vi "Test Square.vi"() -> ()   [LabVIEW 2015, in "SB SubVIs.lvlib"]
uses:
  SB SubVIs.lvlib
  Type Defs/Action Enum.ctl
  Type Defs/Direction Enum.ctl
  Squares/Shawn/Hail/Hail.lvclass
  Read-Only Globals.vi
  Globals (private).vi
  Square/Square.lvclass
  Type Defs/SB Type Defs.lvlib
panel:
  out "Array 2":T1[](array[typedef])
  out "Array":T2[](array[typedef])
  out "Intensity Graph":i32[][](graph)
  in  "stop":bool
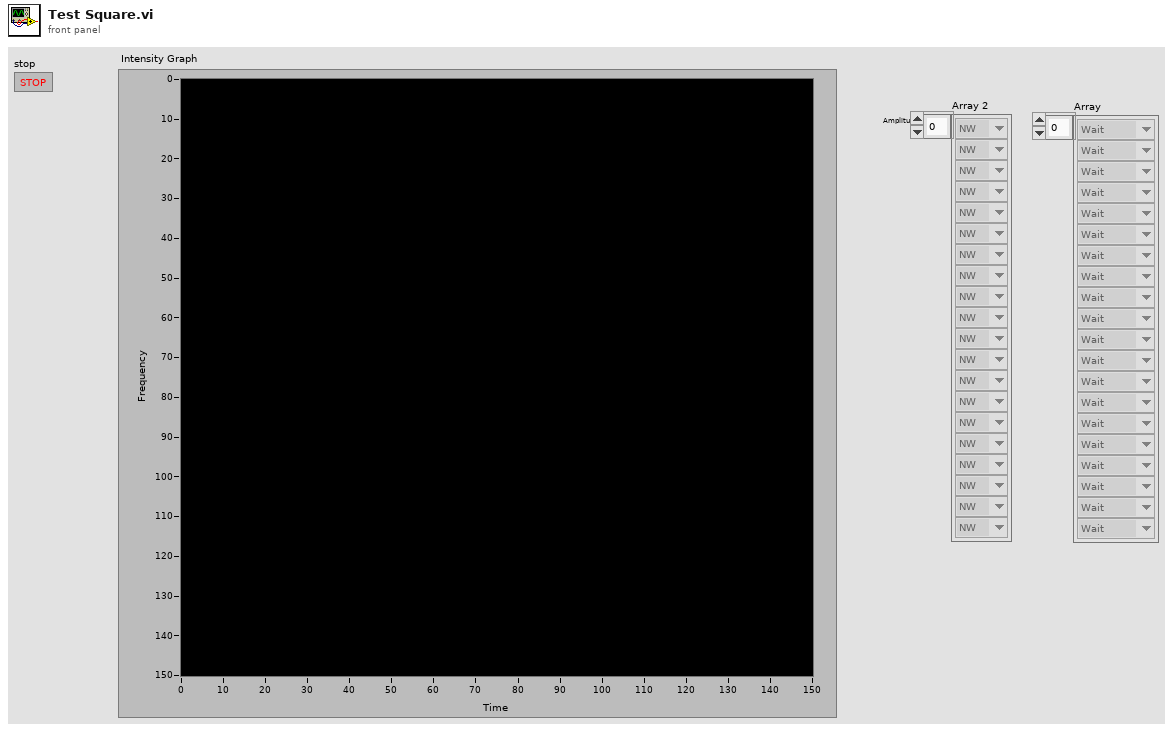
[diagram p1: front panel]
types:
  T1 = typedef "SB Type Defs.lvlib/Direction Enum.ctl" = enum16{"NW", "N", "NE", "E", "SE", "S", "SW", "W"}
  T2 = typedef "SB Type Defs.lvlib/Action Enum.ctl" = enum16{"Wait", "Move", "Attack", "Replicate"}
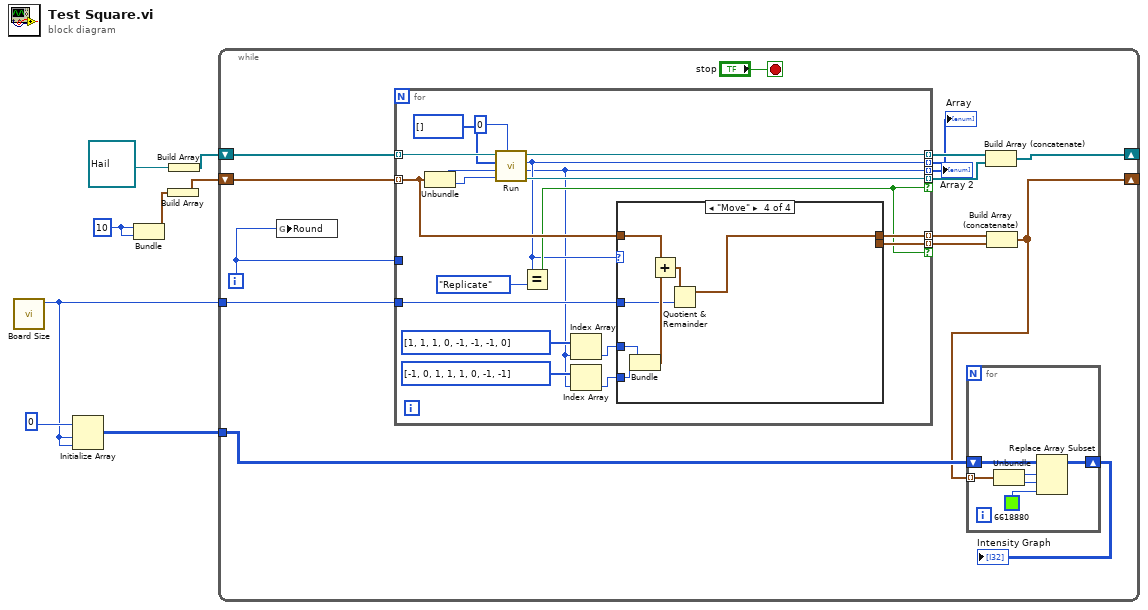
[diagram p0: block diagram]
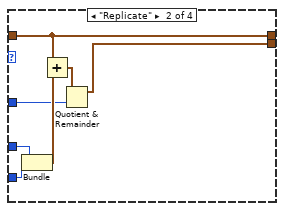
[diagram p3: hidden frame]
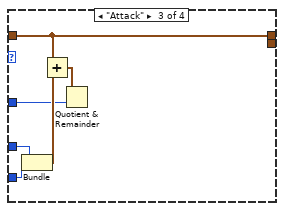
[diagram p4: hidden frame]
diagram:
  w2 = 10
  n1 = call "Board Size.vi"() -> ("Board Size"=w3:i32)  [unwired: 11 in]
  n2 = Initialize Array(0, w3, w3) -> (w1:i32[][])
  n3 = Bundle(w2, w2) -> (w5:cluster{i32, i32})  [unwired: 1 in]
  n4 = Build Array(w5) -> (w6:cluster{i32, i32}[])
  n5 = Build Array(refnum<class "Hail.lvclass"> refnum ("Hail.lvclass")) -> (w8:refnum<class "Hail.lvclass">[])
  n6 = while {
    shift-right: [w20] -> _
    shift-left: w8 -> [w22]
    shift-right: [w11] -> _
    shift-left: w6 -> [w17]
    tunnel: w3 -> [w16]
    tunnel: w1 -> [w13]
    i -> [w23]
    stop <- "stop" stop-if-true
    n7 = global write "Globals (private).vi" "Round"(w23) -> ()
    n8 = for {
      tunnel: w23 -> [_]
      tunnel: w22 -> [w48] mode=indexing
      tunnel: [w47] -> w21 mode=indexing
      tunnel: [w45] -> w19 mode=indexing if=w32
      tunnel: w17 -> [w36] mode=indexing
      tunnel: w16 -> [w34]
      tunnel: [w35] -> w15 mode=indexing
      tunnel: [w33] -> w14 mode=indexing if=w32
      tunnel: [w31] -> w10 mode=indexing
      tunnel: [w30] -> w9 mode=indexing
      n9 = Unbundle(w36) -> (w42:i32, w41:i32)
      n10 = call-dynamic "Run.vi"("Team Index"=0, "Column"=w41, "Row"=w42, "View"=i32[] [], "Square In"=w48) -> ("Replicated"=w45:refnum<class "Square.lvclass">, "Direction"=w30:T1, "Action"=w31:T2, "Square Out"=w47:refnum<class "Square.lvclass">)  [unwired: 3 in]
      n11 = Equal?(x=w31, y=Action_Enum."Replicate") -> (x = y?=w32:bool)
      n12 = Index Array(array=i32[] [1, 1, 1, 0, -1, -1, -1, 0], index=w30) -> (element=w38:i32)
      n13 = Index Array(array=i32[] [-1, 0, 1, 1, 1, 0, -1, -1], index=w30) -> (element=w37:i32)
      n14 = case shown="\"Move\"" w31 {
        tunnel: w38 -> [_ w55 w61 w68]
        tunnel: w37 -> [_ w56 w62 w69]
        tunnel: w36 -> [w49 w51 w57 w63]
        tunnel: [w49 w51 w57 w64] -> w35
        tunnel: w34 -> [_ w52 w58 w65]
        tunnel: [_ w50 _ _] -> w33
        frame "Wait" {
        }
        frame "Replicate" {
          n15 = Bundle("X Loc"=w55, "X Loc"=w56) -> (w54:cluster{"X Loc":i32, "X Loc":i32})  [unwired: 1 in]
          n16 = Add(x=w51, y=w54) -> (x+y=w53:cluster{i32, i32})
          n17 = Quotient & Remainder(x=w53, y=w52) -> (x-y*floor(x/y)=w50:cluster{i32, i32})  [unwired: 1 out]
        }
        frame "Attack" {
          n18 = Bundle("X Loc"=w61, "X Loc"=w62) -> (w60:cluster{"X Loc":i32, "X Loc":i32})  [unwired: 1 in]
          n19 = Add(x=w57, y=w60) -> (x+y=w59:cluster{i32, i32})
          n20 = Quotient & Remainder(x=w59, y=w58) -> ()  [unwired: 2 out]
        }
        frame "Move" {
          n21 = Bundle("X Loc"=w68, "X Loc"=w69) -> (w67:cluster{"X Loc":i32, "X Loc":i32})  [unwired: 1 in]
          n22 = Add(x=w63, y=w67) -> (x+y=w66:cluster{i32, i32})
          n23 = Quotient & Remainder(x=w66, y=w65) -> (x-y*floor(x/y)=w64:cluster{i32, i32})  [unwired: 1 out]
        }
      }
    }
    "Array" <- w10
    "Array 2" <- w9
    n24 = Build Array (concatenate)(w21, w19) -> (w20:refnum<class "Square.lvclass">[])
    n25 = Build Array (concatenate)(w15, w14) -> (w11:cluster{i32, i32}[])
    n26 = for {
      shift-right: [w28] -> w12
      shift-left: w13 -> [w29]
      tunnel: w11 -> [w26] mode=indexing
      n27 = Unbundle(w26) -> (w25:i32, w24:i32)
      n28 = Replace Array Subset(array=w29, new element=u32 6618880, index (row)=w25, index (col)=w24) -> (w28:i32[][])
    }
    "Intensity Graph" <- w12
  }
